vi "Get Current.vi"(0 "Tree Reference In":refnum<vi>, 5 "error in (no error)":errorcluster, 9 "Column # (0)":i32) -> (14 "Tree Reference Out":refnum<vi>, 16 "Current Tag":string, 17 "Current Text":string, 19 "error out":errorcluster)   [LabVIEW 2012, in "QuickVIew.lvlib"]
doc: "Returns the tag of the currently selected item in the tree. If there is no item selected an empty string is returned."
uses:
  QuickVIew.lvlib
panel:
  # "VI INPUTS"
  # "VI OUTPUTS"
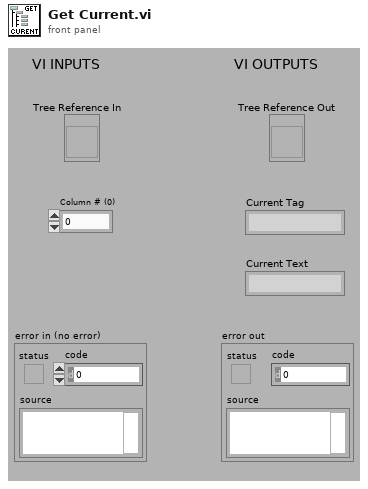
[diagram p1: front panel]
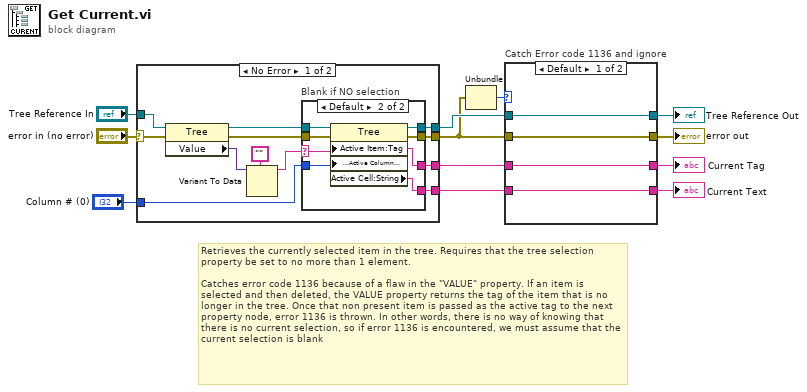
[diagram p0: block diagram]
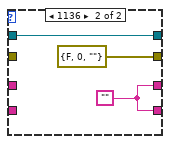
[diagram p2: hidden frame]
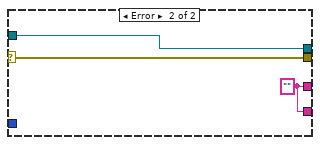
[diagram p4: hidden frame]
diagram:
  # "Retrieves the currently selected item in the tree. Requires that the tree selection property be set to no more than 1 element. \n\nCatches error code 1136 because of a flaw in the \"VALUE\" property. If an item is selected and then deleted, the VALUE property returns the tag of the item that is no longer in the tree. Once that non present item is passed as the active tag to the next property node, error 1136 is thrown. In other words, there is no way of knowing that there is no current selection, so if error 1136 is encountered, we must assume that the current selection is blank"
  n1 = case shown="No Error" "error in (no error)" {
    selector: "error in (no error)" -> [w14 w36]
    tunnel: "Tree Reference In" -> [w24 w37]
    tunnel: [w18 w37] -> w11
    tunnel: [w17 w35] -> w8
    tunnel: [w20 w36] -> w2
    tunnel: [w15 w35] -> w9
    tunnel: "Column # (0)" -> [w13 _]
    frame No Error {
      n2 = property class="Tree"(reference=w24, error in=w14) -> (reference out=w19:refnum<vi>, error out=w23:errorcluster, "Value"=w22:variant)
      n3 = Variant To Data(type="", Variant=w22) -> (data=w16:string)  [unwired: 1 in, 1 out]
      n4 = case "Blank if NO selection" shown="Default" w16 {
        selector: w16 -> [w26 w29]
        tunnel: w23 -> [w25 w34]
        tunnel: [w25 w33] -> w20
        tunnel: w19 -> [w27 w32]
        tunnel: [w27 w31] -> w18
        tunnel: [w26 w30] -> w17
        tunnel: [w26 w29] -> w15
        tunnel: w13 -> [_ w28]
        frame "" {
        }
        frame Default {
          n5 = property class="Tree"(reference=w32, error in=w34, "Active Item:Tag"=w29, "Active Cell:Active Column Number"=w28) -> (reference out=w31:refnum<vi>, error out=w33:errorcluster, "Active Cell:String"=w30:string)
        }
      }
    }
    frame Error {
      w35 = ""
    }
  }
  n6 = Unbundle(w2) -> ("code"=w3:i32)  [unwired: 2 out]
  n7 = case "Catch Error code 1136 and ignore" shown="Default" w3 {
    tunnel: w11 -> [w41 w44]
    tunnel: w9 -> [w39 _]
    tunnel: w8 -> [w38 _]
    tunnel: [w41 w44] -> w7
    tunnel: [w39 w43] -> w6
    tunnel: [w38 w43] -> w5
    tunnel: [w40 errorcluster {"status"=FALSE, "code"=0, "source"=""}] -> w4
    tunnel: w2 -> [w40 _]
    frame Default {
    }
    frame 1136 {
      w43 = ""
    }
  }
  "error out" <- w4
  "Tree Reference Out" <- w7
  "Current Tag" <- w6
  "Current Text" <- w5
